vi "StartAcquisition.vi"(0 "Communication in":refnum<class "Microscope.lvclass">, 5 "Exposure":i32=100, 7 "Frames":i32=100, 9 "Interval":i32=100, 11 "error in (no error)":errorcluster) -> (4 "Communication out":refnum<class "Microscope.lvclass">, 15 "error out":errorcluster)   [LabVIEW 2020]
uses:
  Microscope.lvclass
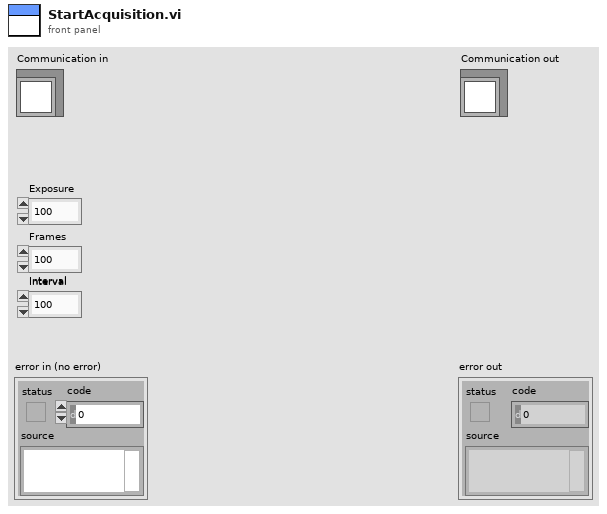
[diagram p1: front panel]
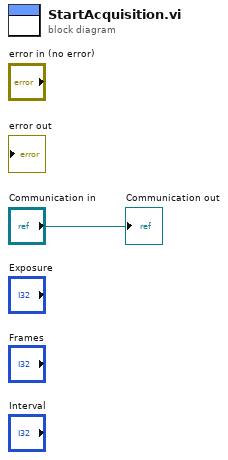
[diagram p0: block diagram]
diagram:
  "Communication out" <- "Communication in"
